vi "Periodic Tasks.vi"(8 "error in":errorcluster) -> ()   [LabVIEW 2015]
doc: "This VI runs in parallel to other tasks. It can contain as many user-defined periodic loops as you need. These can carry out PID or other sorts of timed response."
uses:
  <vilib>/Rock Robotics/WPI/Utilities/WPI_GetSetVariantRefNum.vi
  Robot Global Data.vi
  <vilib>/Rock Robotics/Network Tables/NT Write Number.vi
  <vilib>/Rock Robotics/Network Tables/NT Write Boolean.vi
panel:
  in  "Simulated Hall Effect Sensor":bool
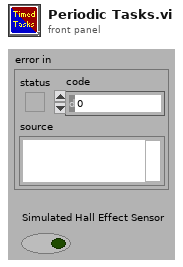
[diagram p1: front panel]
types:
  T1 = typedef "WPI_JoystickDevRef.ctl" = cluster{"Device":T2}
  T2 = typedef "WPI_JoystickDeviceEnum.ctl" = enum16{"USB 0", "USB 1", "USB 2", "USB 3", "USB 4", "USB 5"}
  T3 = typedef "WPI_RobotDriveDevRef.ctl" = cluster{"DevStatus":errorcluster, "Motors[]":T4[], "Square Inputs":bool, "Max Output":dbl}
  T4 = typedef "WPI_MotorControlDeviceRef.ctl" = cluster{"DeviceStatus":errorcluster, "Type":T5, "PWM":cluster{"PWM Channel":T6, "DeadBand":T7}, "CAN":cluster{"Device Number":u8, "Control Mode":T8, "Semaphore":T9, "Max Vout":dbl, "TalonSRX Control Mode":T10}, "Invert":bool}
  T5 = typedef "WPI_MotorControlType.ctl" = enum16{"PWM", "CAN", "CANTalonSRX"}
  T6 = typedef "FPGA_DIOPWMChannel.ctl" = enum8{"PWM 0", "PWM 1", "PWM 2", "PWM 3", "PWM 4", "PWM 5", "PWM 6", "PWM 7", "PWM 8", "PWM 9", "PWM MXP 0", "PWM MXP 1", "PWM MXP 2", "PWM MXP 3", "PWM MXP 4", "PWM MXP 5", "PWM MXP 6", "PWM MXP 7", "PWM MXP 8", "PWM MXP 9", "Invalid"}
  T7 = typedef "WPI_PWMDeadband.ctl" = cluster{"Name":string, "maxPositivePwm":i32, "minPositivePwm":i32, "centerPwm":i32, "maxNegativePwm":i32, "minNegativePwm":i32, "angularRange":u16}
  T8 = typedef "WPI_CANJaguar_ControlMode.ctl" = enum8{"Percent VBus", "Current", "Speed", "Position", "Voltage"}
  T9 = typedef "Semaphore RefNum" = refnum<k1>
  T10 = typedef "WPI_CANTalonSRX_APIControlMode.ctl" = enum8{"Percent VBus", "Speed", "Position", "Slave", "Unchanged / Invalid", "Voltage Compensation", "Current", "Motion Profile"}
  T11 = cluster{"JoystickDevRef":T1, "JoystickDevRef":T1, "RobotDriveDevRef":T3}
  T12 = typedef "WPI_PotentiometerDevRef.ctl" = cluster{"DevStatus":errorcluster, "Analog Channel":T13, "Invert Output":bool}
  T13 = typedef "FPGA_AIChannel.ctl" = enum8{"AI 0", "AI 1", "AI 2", "AI 3", "AI MXP 0", "AI MXP 1", "AI MXP 2", "AI MXP 3", "Invalid"}
  T14 = typedef "WPI_DigitalInputDevRef.ctl" = cluster{"DevStatus":errorcluster, "DIO Channel":T15}
  T15 = typedef "FPGA_DIOChannel.ctl" = enum8{"DIO 0", "DIO 1", "DIO 2", "DIO 3", "DIO 4", "DIO 5", "DIO 6", "DIO 7", "DIO 8", "DIO 9", "DIO MXP 0", "DIO MXP 1", "DIO MXP 2", "DIO MXP 3", "DIO MXP 4", "DIO MXP 5", "DIO MXP 6", "DIO MXP 7", "DIO MXP 8", "DIO MXP 9", "DIO MXP 10", "DIO MXP 11", "DIO MXP 12", "DIO MXP 13", "DIO MXP 14", "DIO MXP 15", "Invalid"}
  T16 = typedef "IMUDevRef.ctl" = cluster{"DevStatus":errorcluster, "Gyro Address":u8, "Gyro Range":u8, "Mean Rates":cluster{"Xmo":dbl, "Ymo":dbl, "Zmo":dbl}, "StdDev Rates":cluster{"Xsdo":dbl, "Ysdo":dbl, "Zsdo":dbl}, "Fast":bool, "Reset":bool, "Accel Address":u8, "Accel Range":u8, "Accel Scale":cluster{"Xscale":dbl, "Yscale":dbl, "Zscale":dbl}, "Mag Address":u8, "Mag Range":u8, "G Sense":bool, "A Sense":bool, "M Sense":bool, "Accel Offset":cluster{"Xzero":dbl, "Yzero":dbl, "Zzero":dbl}, "Motion Thresh":dbl, "Mag Scale":cluster{"Xscale":dbl, "Yscale":dbl, "Zscale":dbl}, "Mag Offset":cluster{"Xzero":dbl, "Yzero":dbl, "Zzero":dbl}, "I2C Bus":T17, "Handle":i32, "Anomaly Thresh":dbl, "Local Mag":dbl}
  T17 = typedef "i2c_bus.ctl" = enum16{"I2C On-Board", "I2C MXP", "Invalid"}
  T18 = typedef "WPI_SwitchDevRef.ctl" = cluster{"DevStatus":errorcluster, "DIO Channel":T15, "CntIndex":T19, "Normally Closed":bool}
  T19 = typedef "FPGA_CounterCtrSystemIndex.ctl" = enum8{"Ctr 0", "Ctr 1", "Ctr 2", "Ctr 3", "Ctr 4", "Ctr 5", "Ctr 6", "Ctr 7", "Invalid"}
  T20 = typedef "Gyro.ctl" = cluster{"Xrate":dbl, "Yrate":dbl, "Zrate":dbl, "Xdeg":dbl, "Ydeg":dbl, "Zdeg":dbl, "dt":dbl}
  T21 = typedef "WPI_GyroDevRef.ctl" = cluster{"DevStatus":errorcluster, "Analog Channel":T13, "Offset":dbl, "Gain (VoltsPerDegree/Second)":dbl, "Gyro Type":enum16{"Analog", "XRS450"}, "Handle":i32, "SPI Bus":T22, "Device Found":bool, "Sample Rate":dbl, "Calibrate On Open":bool}
  T22 = typedef "spi_bus.ctl" = enum16{"SPI On-Board, CS0", "SPI On-Board, CS1", "SPI On-Board, CS2", "SPI On-Board, CS3", "SPI MXP", "Invalid"}
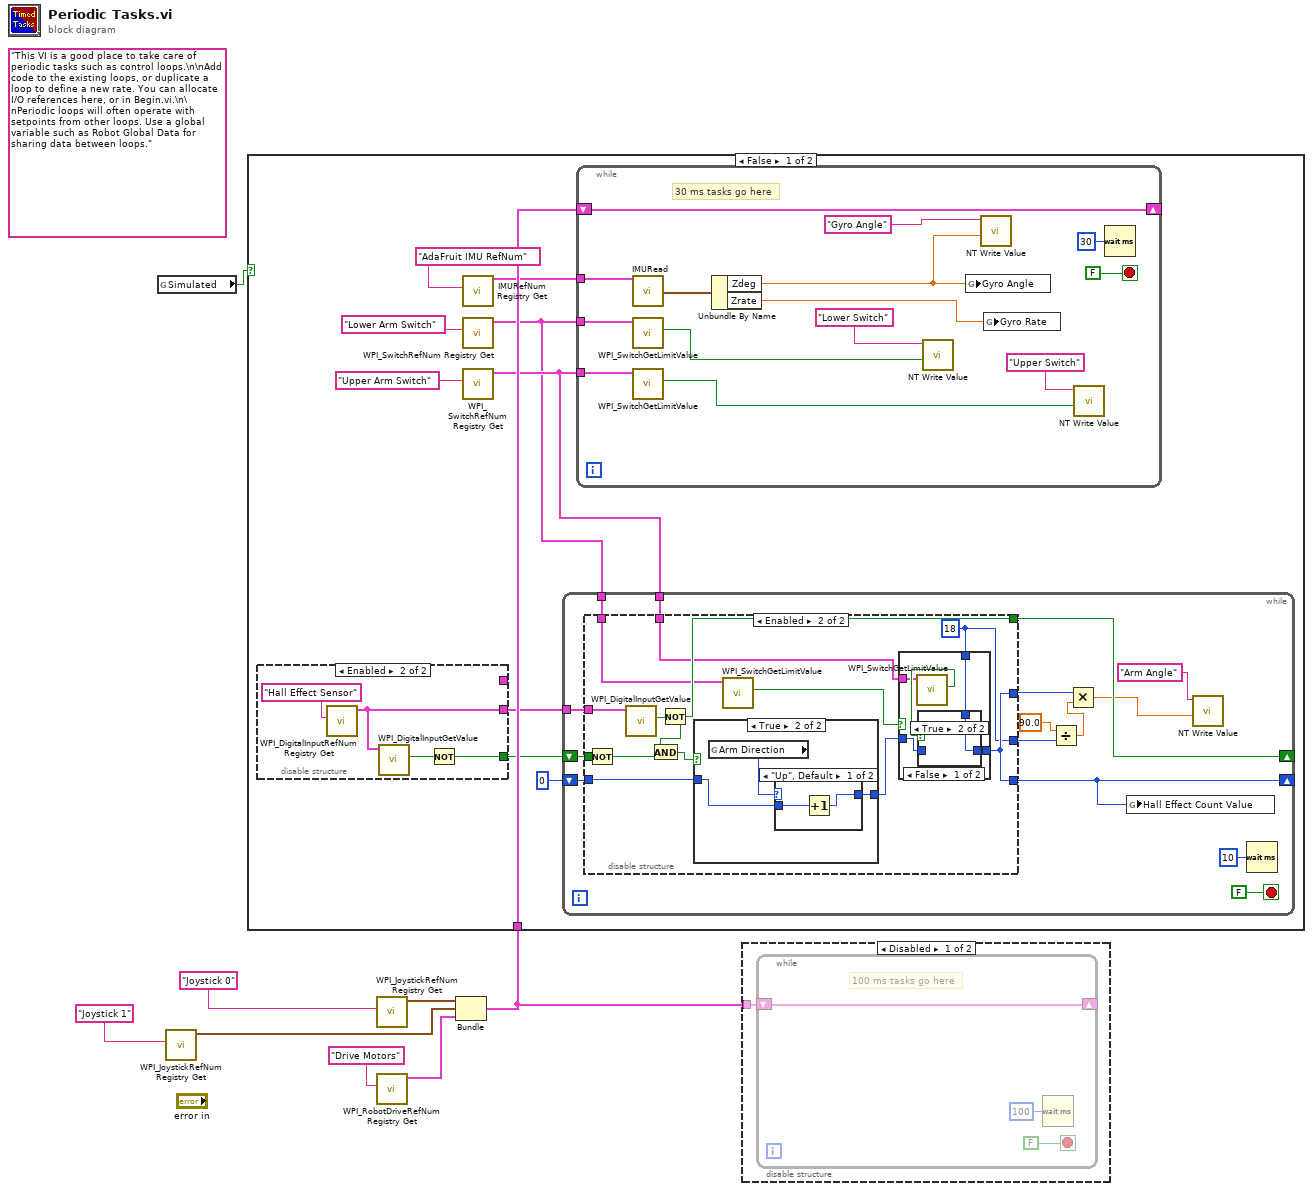
[diagram p0: block diagram]
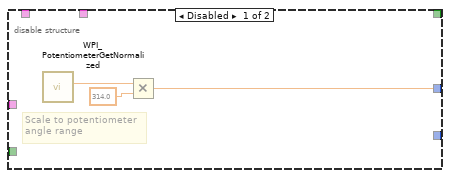
[diagram p2: hidden frame]
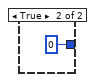
[diagram p4: hidden frame]
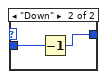
[diagram p6: hidden frame]
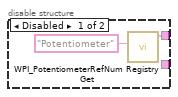
[diagram p7: hidden frame]
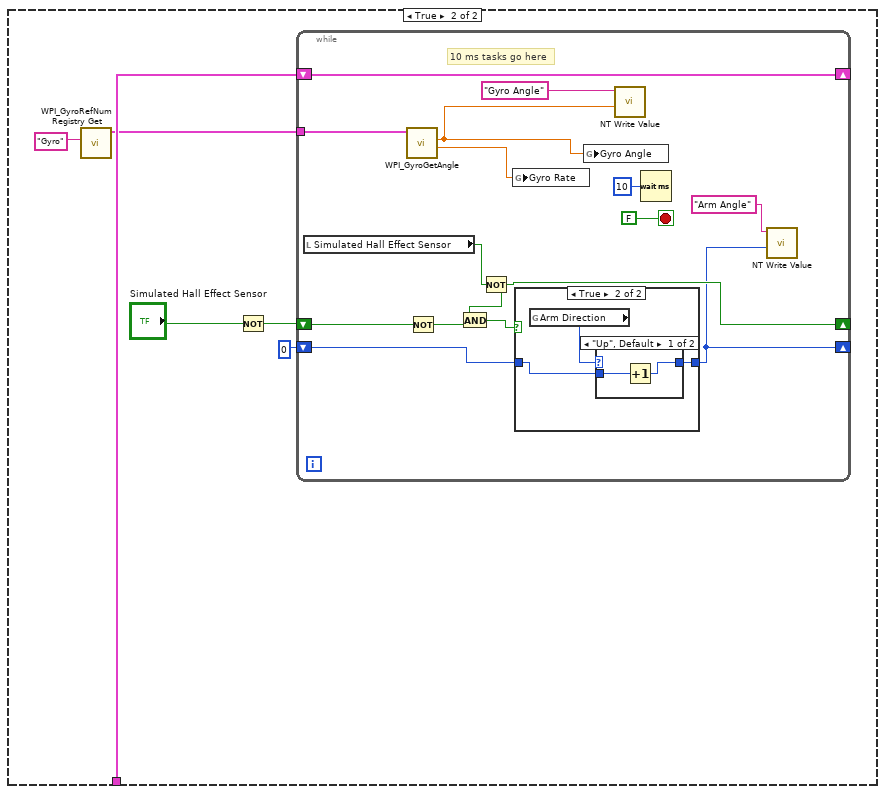
[diagram p8: hidden frame]
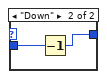
[diagram p10: hidden frame]
diagram:
  (unwired) "This VI is a good place to take care of periodic tasks such as control loops.\n\nAdd code to the existing loops, or duplicate a loop to define a new rate. You can allocate I/O references here, or in Begin.vi.\n\nPeriodic loops will often operate with setpoints from other loops. Use a global variable such as Robot Global Data for sharing data between loops."
  n1 = global read "Robot Global Data.vi" "Simulated"() -> (w1:bool)
  n2 = call <vilib>:"WPI_JoystickRefNum Registry Get.vi"("refnum name"="Joystick 1") -> ("JoystickDevRef"=w2:T1)  [unwired: 1 in, 9 out]
  n3 = call <vilib>:"WPI_JoystickRefNum Registry Get.vi"("refnum name"="Joystick 0") -> ("JoystickDevRef"=w6:T1)  [unwired: 1 in, 9 out]
  n4 = call <vilib>:"WPI_RobotDriveRefNum Registry Get.vi"("refnum name"="Drive Motors") -> ("RobotDriveDevRef"=w3:T3)  [unwired: 1 in, 9 out]
  n5 = Bundle("JoystickDevRef"=w6, "JoystickDevRef"=w2, "RobotDriveDevRef"=w3) -> (w5:T11)  [unwired: 1 out]
  n6 = case shown="False" w1 {
    tunnel: w5 -> [w18 w91]
    frame False {
      n7 = disable-structure shown="Enabled" {
        disable-tunnel: [w67 _] -> _
        disable-tunnel: [_ w70] -> w13
        disable-tunnel: [_ w68] -> w12
        frame Disabled {
          n8 = call <vilib>:"WPI_PotentiometerRefNum Registry Get.vi"("refnum name"="Potentiometer") -> ("PotDevRef"=w67:T12)  [unwired: 9 in, 1 out]
        }
        frame Enabled {
          n9 = call <vilib>:"WPI_DigitalInputRefNum Registry Get.vi"("refnum name"="Hall Effect Sensor") -> ("DigitalInputDevRef"=w70:T14)  [unwired: 9 in, 1 out]
          n10 = call <vilib>:"WPI_DigitalInputGetValue.vi"("DigitalInputDevRef"=w70) -> ("Value"=w69:bool)  [unwired: 8 in, 2 out]
          n11 = Not(x=w69) -> (.not. x?=w68:bool)
        }
      }
      n12 = call "IMURefNum Registry Get.vi"("refnum name"="AdaFruit IMU RefNum") -> ("AdaIMUDevRef Out"=w16:T16)  [unwired: 9 in, 1 out]
      n13 = call <vilib>:"WPI_SwitchRefNum Registry Get.vi"("refnum name"="Lower Arm Switch") -> ("SwitchDevRef"=w9:T18)  [unwired: 9 in, 1 out]
      n14 = call <vilib>:"WPI_SwitchRefNum Registry Get.vi"("refnum name"="Upper Arm Switch") -> ("SwitchDevRef"=w10:T18)  [unwired: 9 in, 1 out]
      n15 = while {
        tunnel: w13 -> [w32]
        shift-right: [w29] -> _
        shift-left: w12 -> [w31]
        shift-right: [w22] -> _
        shift-left: 0 -> [w30]
        tunnel: w10 -> [w21]
        tunnel: w9 -> [w20]
        stop <- FALSE stop-if-true
        n16 = disable-structure shown="Enabled" {
          disable-tunnel: [w34 w41] -> w26
          disable-tunnel: w32 -> [_ w49]
          disable-tunnel: w31 -> [_ w48]
          disable-tunnel: w30 -> [_ w45]
          disable-tunnel: [_ w41] -> w22
          disable-tunnel: [_ w43] -> w29
          disable-tunnel: w21 -> [_ w37]
          disable-tunnel: w20 -> [_ w40]
          disable-tunnel: [_ w38] -> w19
          frame Disabled {
            # "Scale to potentiometer\nangle range"
            n17 = call <vilib>:"WPI_PotentiometerGetNormalized.vi"() -> ("Normalized Value"=w36:dbl)  [unwired: 9 in, 2 out]
            n18 = Multiply(x=w36, y=314.0) -> (x*y=w34:dbl)
          }
          frame Enabled {
            w38 = 18 ("y")
            n19 = Not(x=w48) -> (.not. x?=w47:bool)
            n20 = call <vilib>:"WPI_DigitalInputGetValue.vi"("DigitalInputDevRef"=w49) -> ("Value"=w44:bool)  [unwired: 8 in, 2 out]
            n21 = Not(x=w44) -> (.not. x?=w43:bool)
            n22 = And(x=w43, y=w47) -> (x .and. y?=w46:bool)
            n23 = case shown="True" w46 {
              tunnel: w45 -> [w58 w60]
              tunnel: [w58 w59] -> w42
              frame False {
              }
              frame True {
                n24 = global read "Robot Global Data.vi" "Arm Direction"() -> (w61:enum16{"Up", "Down"})
                n25 = case shown="\"Up\", Default" w61 {
                  tunnel: w60 -> [w63 w65]
                  tunnel: [w62 w64] -> w59
                  frame "Up", Default {
                    n26 = Increment(x=w63) -> (x+1=w62:i32)
                  }
                  frame "Down" {
                    n27 = Decrement(x=w65) -> (x-1=w64:i32)
                  }
                }
              }
            }
            n28 = call <vilib>:"WPI_SwitchGetLimitValue.vi"("SwitchDevRef"=w40) -> ("Switch Pressed"=w39:bool)  [unwired: 8 in, 2 out]
            n29 = case shown="False" w39 {
              tunnel: w42 -> [w54 _]
              tunnel: [w53 0 ("y")] -> w41
              tunnel: w38 -> [w52 _]
              tunnel: w37 -> [w50 _]
              frame False {
                n30 = call <vilib>:"WPI_SwitchGetLimitValue.vi"("SwitchDevRef"=w50) -> ("Switch Pressed"=w51:bool)  [unwired: 8 in, 2 out]
                n31 = case shown="True" w51 {
                  tunnel: w54 -> [w55 _]
                  tunnel: [w55 w56] -> w53
                  tunnel: w52 -> [_ w56]
                  frame False {
                  }
                  frame True {
                  }
                }
              }
              frame True {
              }
            }
          }
        }
        n32 = Divide(x=90.0, y=w19) -> (x/y=w24:dbl)
        n33 = Multiply(x=w26, y=w24) -> (x*y=w23:dbl)
        n34 = global write "Robot Global Data.vi" "Hall Effect Count Value"(w22) -> ()
        n35 = call-poly <vilib>:"NT Write Value.vi"("Numeric"=w23, "Name"="Arm Angle") -> ()  [unwired: 9 in, 1 out]
        n36 = Wait (ms)(milliseconds to wait=u32 10) -> ()  [unwired: 1 out]
      }
      n37 = while {
        shift-right: [w83] -> _
        shift-left: w18 -> [w83]
        tunnel: w16 -> [w82]
        tunnel: w9 -> [w78]
        tunnel: w10 -> [w77]
        stop <- FALSE stop-if-true
        # "30 ms tasks go here"
        n38 = call "IMURead.vi"("AdaIMUDevRef"=w82) -> ("Gyro"=w81:T20)  [unwired: 10 in, 4 out]
        n39 = call <vilib>:"WPI_SwitchGetLimitValue.vi"("SwitchDevRef"=w78) -> ("Switch Pressed"=w74:bool)  [unwired: 8 in, 2 out]
        n40 = call <vilib>:"WPI_SwitchGetLimitValue.vi"("SwitchDevRef"=w77) -> ("Switch Pressed"=w73:bool)  [unwired: 8 in, 2 out]
        n41 = Unbundle By Name(w81) -> ("Zdeg"=w80:dbl, "Zrate"=w72:dbl)
        n42 = call-poly <vilib>:"NT Write Value.vi"("Boolean"=w74, "Name"="Lower Switch") -> ()  [unwired: 9 in, 1 out]
        n43 = global write "Robot Global Data.vi" "Gyro Angle"(w80) -> ()
        n44 = call-poly <vilib>:"NT Write Value.vi"("Numeric"=w80, "Name"="Gyro Angle") -> ()  [unwired: 9 in, 1 out]
        n45 = global write "Robot Global Data.vi" "Gyro Rate"(w72) -> ()
        n46 = call-poly <vilib>:"NT Write Value.vi"("Boolean"=w73, "Name"="Upper Switch") -> ()  [unwired: 9 in, 1 out]
        n47 = Wait (ms)(milliseconds to wait=u32 30) -> ()  [unwired: 1 out]
      }
    }
    frame True {
      n48 = call <vilib>:"WPI_GyroRefNum Registry Get.vi"("refnum name"="Gyro") -> ("GyroDevRef"=w89:T21)  [unwired: 9 in, 1 out]
      n49 = Not(x="Simulated Hall Effect Sensor") -> (.not. x?=w87:bool)
      n50 = while {
        shift-right: [w104] -> _
        shift-left: w91 -> [w104]
        tunnel: w89 -> [w103]
        shift-right: [w93] -> _
        shift-left: 0 -> [w99]
        shift-right: [w98] -> _
        shift-left: w87 -> [w97]
        stop <- FALSE stop-if-true
        # "10 ms tasks go here"
        n51 = local read "Simulated Hall Effect Sensor"() -> (w92:bool)
        n52 = call <vilib>:"WPI_GyroGetAngle.vi"("GyroDevRef"=w103) -> ("Angular Rate"=w100:dbl, "Angle"=w102:dbl)  [unwired: 6 in, 3 out]
        n53 = Not(x=w97) -> (.not. x?=w96:bool)
        n54 = Not(x=w92) -> (.not. x?=w98:bool)
        n55 = And(x=w98, y=w96) -> (x .and. y?=w95:bool)
        n56 = global write "Robot Global Data.vi" "Gyro Rate"(w100) -> ()
        n57 = case shown="True" w95 {
          tunnel: w99 -> [w107 w109]
          tunnel: [w107 w108] -> w93
          frame False {
          }
          frame True {
            n58 = global read "Robot Global Data.vi" "Arm Direction"() -> (w110:enum16{"Up", "Down"})
            n59 = case shown="\"Up\", Default" w110 {
              tunnel: w109 -> [w112 w114]
              tunnel: [w111 w113] -> w108
              frame "Up", Default {
                n60 = Increment(x=w112) -> (x+1=w111:i32)
              }
              frame "Down" {
                n61 = Decrement(x=w114) -> (x-1=w113:i32)
              }
            }
          }
        }
        n62 = global write "Robot Global Data.vi" "Gyro Angle"(w102) -> ()
        n63 = call-poly <vilib>:"NT Write Value.vi"("Numeric"=w102, "Name"="Gyro Angle") -> ()  [unwired: 9 in, 1 out]
        n64 = Wait (ms)(milliseconds to wait=u32 10) -> ()  [unwired: 1 out]
        n65 = call-poly <vilib>:"NT Write Value.vi"("Numeric"=w93, "Name"="Arm Angle") -> ()  [unwired: 9 in, 1 out]
      }
    }
  }
  n66 = disable-structure shown="Disabled" {
    disable-tunnel: w5 -> [w115 _]
    frame Disabled {
      n67 = while {
        shift-right: [w116] -> _
        shift-left: w115 -> [w116]
        stop <- FALSE stop-if-true
        # "100 ms tasks go here"
        n68 = Wait (ms)(milliseconds to wait=u32 100) -> ()  [unwired: 1 out]
      }
    }
    frame Enabled {
    }
  }
